vi "StateNode_Create.vi"(0 "reference":refnum<class "StateNode.lvclass">, 5 "error in (no error)":errorcluster) -> (14 "reference out":refnum<class "StateNode.lvclass">, 19 "error out":errorcluster)   [LabVIEW 2016, in "StateNode.lvclass"]
doc: "Creates and initializes a new StateNode object.\n\nThis object should be destroyed using a StateNode destructor VI or a virtual base class destructor VI.\n\n[GOOP 2.1]"
uses:
  <resource>/Framework/Providers/Open_GDS/UML/StateNode_class/StateNode.lvclass
  C:/Program Files (x86)/National Instruments/LabVIEW 2016/resource/Framework/Providers/Open_GDS/UML/RectangularNode_class/RectangularNode.lvclass
  <resource>/Framework/Providers/Open_GDS/UML/MultiLineString_class/SizeType.ctl
  <resource>/Framework/Providers/Open_GDS/UML/General/Rectangle/Rectangle Rectangle2D.ctl
  <resource>/Framework/Providers/Open_GDS/UML/MultiLineString_class/JustificationType.ctl
  <resource>/Framework/Providers/Open_GDS/UML/MultiLineString_class/MultiLineString.lvclass
  <resource>/Framework/Providers/Open_GDS/UML/RectangularNode_class/RectangularNode.lvclass
panel:
  # "The input reference should only\nbe wired when this method is called\nby a sub class constructor."
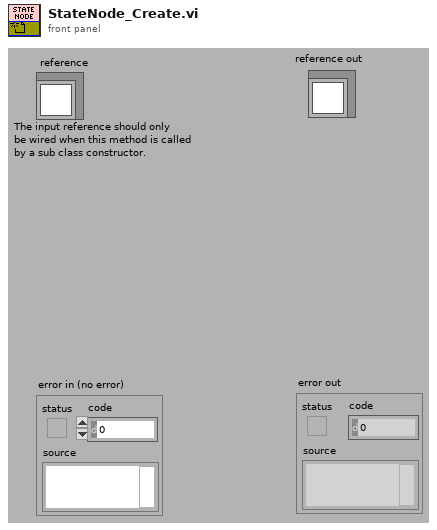
[diagram p1: front panel]
types:
  T1 = typedef "MultiLineString.lvclass/SizeType.ctl" = enum16{"LARGE", "NORMAL", "SMALL"}
  T2 = typedef "MultiLineString.lvclass/JustificationType.ctl" = enum16{"LEFT", "CENTER", "RIGHT"}
  T3 = typedef "Rectangle Rectangle2D.ctl" = cluster{"x":dbl, "y":dbl, "width":dbl, "height":dbl}
  T4 = typedef "StateNode.lvclass/ObjectAttributes.ctl" = cluster{"state":refnum<class "MultiLineString.lvclass">, "action":refnum<class "MultiLineString.lvclass">, "DEFAULT_WIDTH":i32, "DEFAULT_HEIGHT":i32}
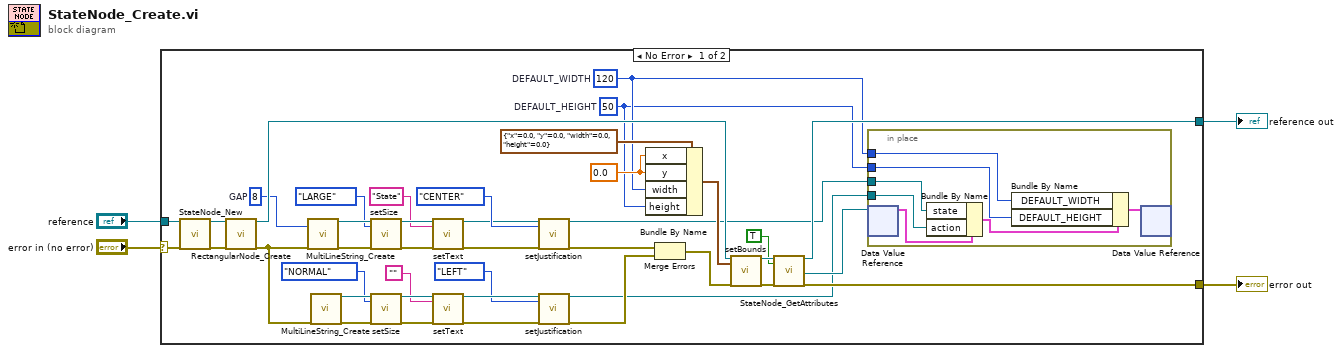
[diagram p0: block diagram]
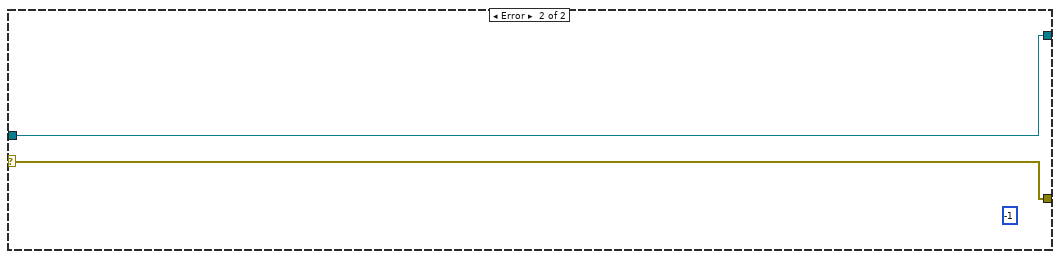
[diagram p2: hidden frame]
diagram:
  n1 = case shown="No Error" "error in (no error)" {
    selector: "error in (no error)" -> [w45 w54]
    tunnel: [w43 w53] -> w4
    tunnel: [w42 w54] -> w3
    tunnel: "reference" -> [w44 w53]
    frame No Error {
      w33 = 0.0 ("x")
      w12 = 8  # GAP
      w5 = 50  # DEFAULT_HEIGHT
      w6 = 120  # DEFAULT_WIDTH
      n2 = call <resource>:"StateNode_New.vi"("reference in"=w44, "error in (no error)"=w45) -> ("reference out"=w32:refnum<class "StateNode.lvclass">, "error out"=w41:errorcluster)  [unwired: 2 in, 14 out]
      n3 = call <resource>:"RectangularNode_Create.vi"("reference"=w32, "error in (no error)"=w41) -> ("reference out"=w36:refnum<class "StateNode.lvclass">, "error out"=w18:errorcluster)  [unwired: 1 in, 15 out]
      n4 = call <resource>:"MultiLineString_Create.vi"("GAP"=w12, "error in (no error)"=w18) -> ("reference out"=w40:refnum<class "MultiLineString.lvclass">, "error out"=w39:errorcluster)  [unwired: 1 in, 15 out]
      n5 = call <resource>:"MultiLineString_Create.vi"("error in (no error)"=w18) -> ("reference out"=w19:refnum<class "MultiLineString.lvclass">, "error out"=w20:errorcluster)  [unwired: 2 in, 15 out]
      n6 = call <resource>:"setSize.vi"("reference"=w40, "size"=SizeType."LARGE", "error in (no error)"=w39) -> ("reference out"=w30:refnum<class "MultiLineString.lvclass">, "error out"=w29:errorcluster)  [unwired: 15 out]
      n7 = call <resource>:"setSize.vi"("reference"=w19, "size"=SizeType."NORMAL", "error in (no error)"=w20) -> ("reference out"=w22:refnum<class "MultiLineString.lvclass">, "error out"=w23:errorcluster)  [unwired: 15 out]
      n8 = call-dynamic "setText.vi"("reference"=w30, "text"="State", "error in (no error)"=w29) -> ("reference out"=w26:refnum<class "MultiLineString.lvclass">, "error out"=w27:errorcluster)  [unwired: 15 in]
      n9 = call-dynamic "setText.vi"("reference"=w22, "text"="", "error in (no error)"=w23) -> ("reference out"=w25:refnum<class "MultiLineString.lvclass">, "error out"=w24:errorcluster)  [unwired: 15 in]
      n10 = call <resource>:"setJustification.vi"("reference"=w26, "justification"=JustificationType."CENTER", "error in (no error)"=w27) -> ("reference out"=w8:refnum<class "MultiLineString.lvclass">, "error out"=w16:errorcluster)  [unwired: 15 out]
      n11 = call <resource>:"setJustification.vi"("reference"=w25, "justification"=JustificationType."LEFT", "error in (no error)"=w24) -> ("reference out"=w7:refnum<class "MultiLineString.lvclass">, "error out"=w14:errorcluster)  [unwired: 15 out]
      n12 = Bundle By Name(cluster=T3 {"x"=0.0, "y"=0.0, "width"=0.0, "height"=0.0} ("bounds"), "x"=w33, "y"=w33, "width"=w6, "height"=w5) -> (w35:T3)
      n13 = Merge Errors(w16, w14) -> (w15:errorcluster)
      n14 = call-dynamic "setBounds.vi"("reference"=w36, "bounds"=w35, "error in (no error)"=w15) -> ("reference out"=w11:refnum<class "StateNode.lvclass">, "error out"=w31:errorcluster)  [unwired: 15 in]
      n15 = call <resource>:"StateNode_GetAttributes.vi"("reference in"=w11, "OnlyGetDvrReference(False)"=TRUE, "error in (no error)"=w31) -> ("reference out"=w43:refnum<class "StateNode.lvclass">, "DataRef"=w9:refnum<data-value>, "error out"=w42:errorcluster)  [unwired: 13 in, 1 out]
      n16 = in-place {
        in-place-border: w8 -> [w51]
        in-place-border: w7 -> [w50]
        in-place-border: w6 -> [w48]
        in-place-border: w5 -> [w47]
        n17 = in-place-dvr #1(w9) -> (w52:T4)  [unwired: 1 out]
        n18 = Bundle By Name(cluster=w52, "state"=w51, "action"=w50) -> (w49:T4)
        n19 = Bundle By Name(cluster=w49, "DEFAULT_WIDTH"=w48, "DEFAULT_HEIGHT"=w47) -> (w46:T4)
        n20 = in-place-dvr #1(w46) -> ()  [unwired: 2 out]
      }
    }
    frame Error {
      (unwired) -1 ("Nr of open handles")
    }
  }
  "error out" <- w3
  "reference out" <- w4
